vi "ewfdfsfds.vi"() -> ()   [LabVIEW 2022 SP3]
panel:
  out "x*y":i32[](array[numeric])
  out "x >= y?":bool[](array[boolean])
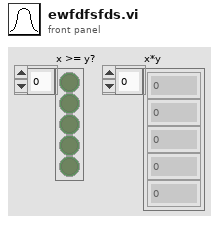
[diagram p1: front panel]
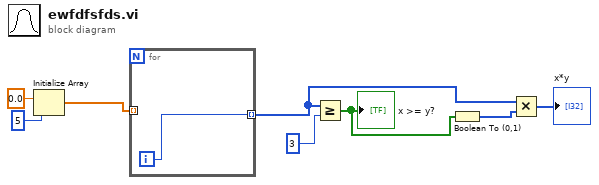
[diagram p0: block diagram]
diagram:
  n1 = Initialize Array(0.0 ("element"), 5 ("dimension size")) -> (w6:dbl[])
  n2 = for {
    tunnel: w6 -> [_] mode=indexing
    tunnel: [w9] -> w2 mode=indexing
    i -> [w9]
  }
  n3 = Greater Or Equal?(x=w2, y=3) -> (x >= y?=w4:bool[])
  "x >= y?" <- w4
  n4 = Boolean To (0,1)(Boolean=w4) -> (0, 1=w3:i16[])
  n5 = Multiply(x=w2, y=w3) -> (x*y=→"x*y":i32[])
